vi "Actor Core.vi"(8 "error in":errorcluster, 11 "Pulse Controller in":refnum<class "Pulse Controller.lvclass">) -> (0 "error out":errorcluster, 3 "Actor out":refnum<class "Actor.lvclass">)   [LabVIEW 2015, in "Pulse Controller.lvclass"]
doc: "(<B>Filename</B>: Actor Framework.lvlib:Actor.lvclass:Actor Core.vi)\n\nReceives messages to the actor, reacts to them, and initiates any error handling that may shut the actor down.\n\nDescendant classes may override this VI to append parallel tasks for the actor to complete while it handles messages. Overrides use the Call Parent Method node."
uses:
  Pulse Controller.lvclass
  <vilib>/ActorFramework/Actor/Actor.lvclass
  Pulse Controller Configuration.ctl
  Measure Controller/Measure Controller.lvclass
panel:
  in  "Configuration":T1={"Pre-trigger duration"=-1.0, "Post-trigger duration"=-1.0, "Open plot after pulse"=FALSE} {"Pre-trigger duration" format="%#_6p"; "Post-trigger duration" format="%#_6p"}
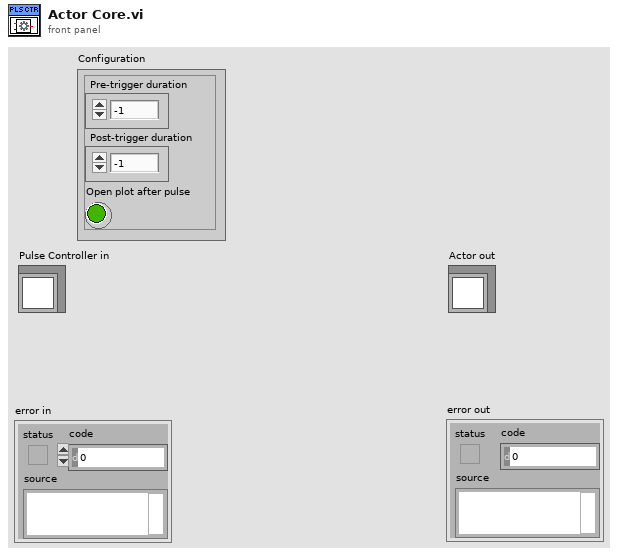
[diagram p1: front panel]
types:
  T1 = typedef "Pulse Controller Configuration.ctl" = cluster{"Pre-trigger duration":dbl, "Post-trigger duration":dbl, "Open plot after pulse":bool}
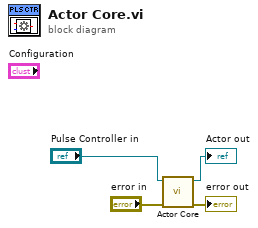
[diagram p0: block diagram]
diagram:
  n1 = call-parent "Actor Core.vi"("error in"="error in", "Measure Object in"="Pulse Controller in") -> ("error out"=→"error out":errorcluster, "Actor out"=→"Actor out":refnum<class "Actor.lvclass">)  [unwired: 8 in]
